vi "im_controller.vi"(6 "Reset":bool, 7 "Parameters":T1={"Stimulus"={"Type"=enum."Off", "Phase"=0.0, "Amplitude"=[0.0, 0.0, 0.0], "Injection point"=enum."Total pose", "Closed loop"=FALSE, "Offset"=[0.0, 0.0, 0.0], "Tip -> world"=TRUE, "Frequency"=0.0, "Length"=0.0}, "Goal Filter A"={"Speedup max"=0.0, "Speedup thresh"=0.15, "Speedup nonlin"=0.0, "Filters"=[]}, "Mode controls"={"Hold"=FALSE, "Cancellation"=FALSE, "Goal filter"=FALSE, "Trigger"=FALSE}, "Manipulator type"=enum."Current piezo", "Manipulator calibration"={"Tool offsets"=[[-0.47364116, -0.25724307, -1.1087934], [0.29673597, -0.25864395, -1.0971603], [-0.04366469, 0.4463568, -1.1035515]], "Tip light calibration"=[[3.2813332, 0.23462732, 0.17832138, -8265.082], [-0.20249099, 2.693321, -0.28150028, -33565.66], [-0.1458117, 0.68216485, 0.8833545, 26862.188], [-1.1202011e-18, 5.861468e-19, 1.7601345e-18, 1.0]], "Handle light calibration"=[[0.0, 0.0, 36200.0]], "Base pivots"=[], "Output pivots"=[[0.0, 0.0, -11360.0]], "Length center"=0.0, "Workspace height"=[], "Workspace diameter"=[0.0, 0.0, 36200.0], "Linearization"=[[0.0, 0.0, 36200.0]], "Stack travel"=400.0, "Saturation pos"=375.0, "Inverse filters"=[]}, "Network"={"Remote Host"="", "Send Status"=FALSE, "Send Port"=50, "Recv Commands"=FALSE, "Recv Port"=0}, "Goal Filter B"={"Speedup max"=0.0, "Speedup thresh"=0.0, "Speedup nonlin"=0.0, "Filters"=[]}, "Cancellation"={"KP"={"XY"=0.0, "Rxy"=0.0, "Z"=0.0, "Rz"=0.0}, "KI"=2.0, "KD"={"XY"=0.0, "Rxy"=0.0, "Z"=0.0, "Rz"=0.0}, "Max vel"=20.0, "Max acc"=61557.0, "Int error limit"=2.0, "RCM gain"=1.0, "Bypass"=FALSE, "Degraded gain"=3.0}, "Transition time"=0.0, "Estimation"={"Link"={"Measure noise"=[], "Process noise"=[], "Alt process noise"=[], "Alt turnoff cycles"=20, "Innovation limit"=[], "Residue threshold"=0.0, "Enable"=FALSE}, "Handle"={"Measure noise"=[], "Process noise"=[], "State limits"=[], "Innovation limit"=[], "Prediction Lookahead"=0.0, "Enable"=FALSE}}} {"Transition time" format="%_3f"; "Cancellation"."Degraded gain" min=0 max=1 step=0.1 format="%#_3p"; "Cancellation"."RCM gain" min=0 max=1 step=0.1 format="%#_3p"; "Cancellation"."KD"."Rz" min=0 max=1 step=0.1 format="%#_3p"; "Cancellation"."KD"."Rxy" min=0 max=1 step=0.1 format="%#_3p"; "Cancellation"."KD"."Z" min=0 max=1 step=0.1 format="%#_3p"; "Cancellation"."KD"."XY" min=0 max=1 step=0.1 format="%#_3p"; "Cancellation"."KI" min=0 max=1 step=0.01 format="%#_3p"; "Cancellation"."KP"."Rz" min=0 max=1 step=0.1 format="%#_3p"; "Cancellation"."KP"."Rxy" min=0 max=1 step=0.1 format="%#_3p"; "Cancellation"."KP"."Z" min=0 max=1 step=0.1 format="%#_3p"; "Cancellation"."KP"."XY" min=0 max=1 step=0.1 format="%#_3p"; "Cancellation"."Max acc" format="%#_3p"; "Goal Filter B"."Filters"."V limit range" format="%_3p"; "Goal Filter B"."Filters"."V limit" format="%_3p"; "Goal Filter B"."Filters"."Upper Q" format="%_3f"; "Goal Filter B"."Filters"."Upper Fc" format="%_3p"; "Goal Filter B"."Filters"."Lower Q" format="%_3f"; "Goal Filter B"."Filters"."Scale factor" format="%_3f"; "Goal Filter B"."Filters"."Lower Fc" format="%_3p"; "Goal Filter B"."Speedup nonlin" format="%_3p"; "Goal Filter B"."Speedup thresh" format="%_3p"; "Goal Filter B"."Speedup max" format="%_3p"; "Manipulator calibration"."Saturation pos" format="%#.1f"; "Manipulator calibration"."Stack travel" format="%#.1f"; "Manipulator calibration"."Output pivots" format="%#_6f"; "Manipulator calibration"."Base pivots" format="%#_6f"; "Manipulator calibration"."Handle light calibration" format="%#.1f"; "Manipulator calibration"."Tip light calibration" format="%#.1f"; "Goal Filter A"."Filters"."V limit range" format="%_3p"; "Goal Filter A"."Filters"."V limit" format="%_3p"; "Goal Filter A"."Filters"."Upper Q" format="%_3f"; "Goal Filter A"."Filters"."Upper Fc" format="%_3p"; "Goal Filter A"."Filters"."Lower Q" format="%_3f"; "Goal Filter A"."Filters"."Scale factor" format="%_3f"; "Goal Filter A"."Filters"."Lower Fc" format="%_3p"; "Goal Filter A"."Speedup nonlin" format="%_3p"; "Goal Filter A"."Speedup thresh" format="%_3p"; "Goal Filter A"."Speedup max" format="%_3p"; "Stimulus"."Length" min=0.0 max=100.0 step=100.0 format="%#_4p"; "Stimulus"."Frequency" min=0.0 step=100.0 format="%#_4g"; "Stimulus"."Offset" format="%#_3p"; "Stimulus"."Amplitude" format="%#_3p"; "Stimulus"."Phase" min=-180.0 max=360.0 step=100.0 format="%#.2f"}, 8 "Manipulator status":sgl[](array[numeric]), 10 "Stack error in":sgl[](array[numeric])) -> (4 "Saturation":bool, 5 "Output":sgl[](array[numeric]))   [LabVIEW 2013]
uses:
  testing/injection_point.ctl
  testing/stimulus.ctl
  testing/mode_conrols.ctl
  testing/Micron params.ctl
  asap/labview/testing/probe_calibration.ctl
  host/network_params.ctl
  testing/manipulator_cal.ctl
  filtering/goal_loop_parms.ctl
  decoupled_gain.ctl
  sq_control_params.ctl
  estimation_controls.ctl
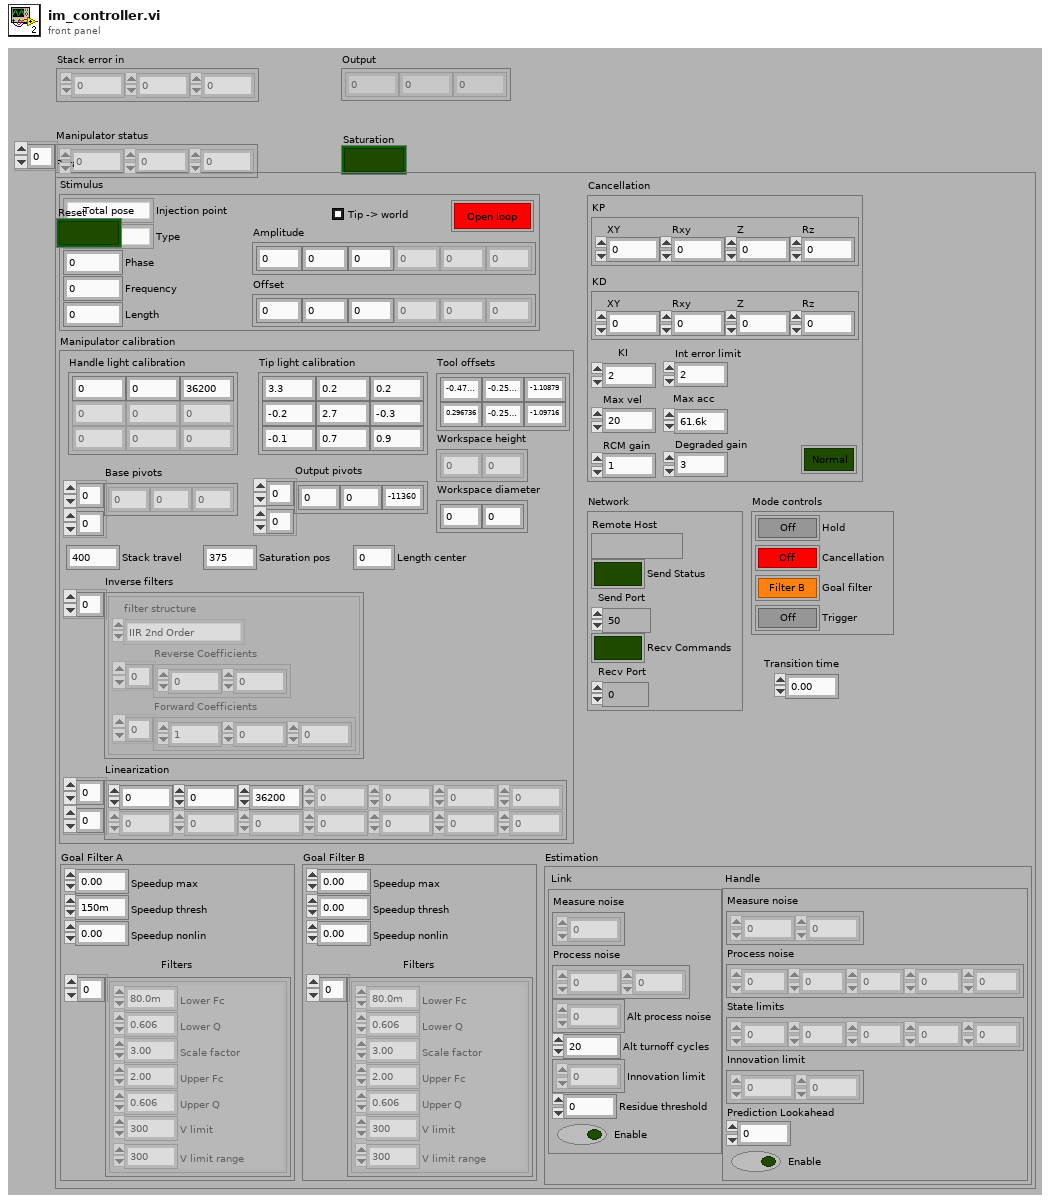
[diagram p1: front panel]
types:
  T1 = typedef "Micron params.ctl" = cluster{"Stimulus":T2, "Goal Filter A":T4, "Mode controls":T5, "Manipulator type":enum16{"Current piezo", "Voltage piezo"}, "Manipulator calibration":T6, "Network":T8, "Goal Filter B":T4, "Cancellation":T9, "Transition time":sgl, "Estimation":T11}
  T2 = typedef "stimulus.ctl" = cluster{"Type":enum16{"Off", "Step", "Sine", "Triangle", "Arbitrary"}, "Phase":dbl, "Amplitude":sgl[], "Injection point":T3, "Closed loop":bool, "Offset":sgl[], "Tip -> world":bool, "Frequency":dbl, "Length":dbl}
  T3 = typedef "injection_point.ctl" = enum16{"Total pose", "V limiter", "Goal ", "Link position", "KF link position", "Inverse kin", "Link goal", "Link error", "Controller", "Output", "Drive", "Light"}
  T4 = typedef "goal_loop_parms.ctl" = cluster{"Speedup max":sgl, "Speedup thresh":sgl, "Speedup nonlin":sgl, "Filters":cluster{"Lower Fc":sgl, "Lower Q":sgl, "Scale factor":sgl, "Upper Fc":sgl, "Upper Q":sgl, "V limit":sgl, "V limit range":sgl}[]}
  T5 = typedef "mode_conrols.ctl" = cluster{"Hold":bool, "Cancellation":bool, "Goal filter":bool, "Trigger":bool}
  T6 = typedef "manipulator_cal.ctl" = cluster{"Tool offsets":sgl[][], "Tip light calibration":T7, "Handle light calibration":T7, "Base pivots":sgl[][], "Output pivots":sgl[][], "Length center":sgl, "Workspace height":sgl[], "Workspace diameter":sgl[], "Linearization":sgl[][], "Stack travel":sgl, "Saturation pos":sgl, "Inverse filters":cluster{"filter structure":enum32{"IIR 2nd Order", "IIR 4th Order"}, "Reverse Coefficients":dbl[], "Forward Coefficients":dbl[]}[]}
  T7 = typedef "probe_calibration.ctl" = sgl[][]
  T8 = typedef "network_params.ctl" = cluster{"Remote Host":string, "Send Status":bool, "Send Port":u16, "Recv Commands":bool, "Recv Port":u16}
  T9 = typedef "sq_control_params.ctl" = cluster{"KP":T10, "KI":sgl, "KD":T10, "Max vel":sgl, "Max acc":sgl, "Int error limit":sgl, "RCM gain":sgl, "Bypass":bool, "Degraded gain":sgl}
  T10 = typedef "decoupled_gain.ctl" = cluster{"XY":sgl, "Rxy":sgl, "Z":sgl, "Rz":sgl}
  T11 = typedef "estimation_controls.ctl" = cluster{"Link":cluster{"Measure noise":dbl[], "Process noise":dbl[], "Alt process noise":dbl[], "Alt turnoff cycles":i32, "Innovation limit":dbl[], "Residue threshold":dbl, "Enable":bool}, "Handle":cluster{"Measure noise":dbl[], "Process noise":dbl[], "State limits":dbl[], "Innovation limit":dbl[], "Prediction Lookahead":sgl, "Enable":bool}}
  T12 = cluster{"XY":dbl, "Rxy":dbl, "Z":dbl, "Rz":dbl}[]
  T13 = cluster{"XY":bool, "Rxy":bool, "Z":bool, "Rz":bool}[]
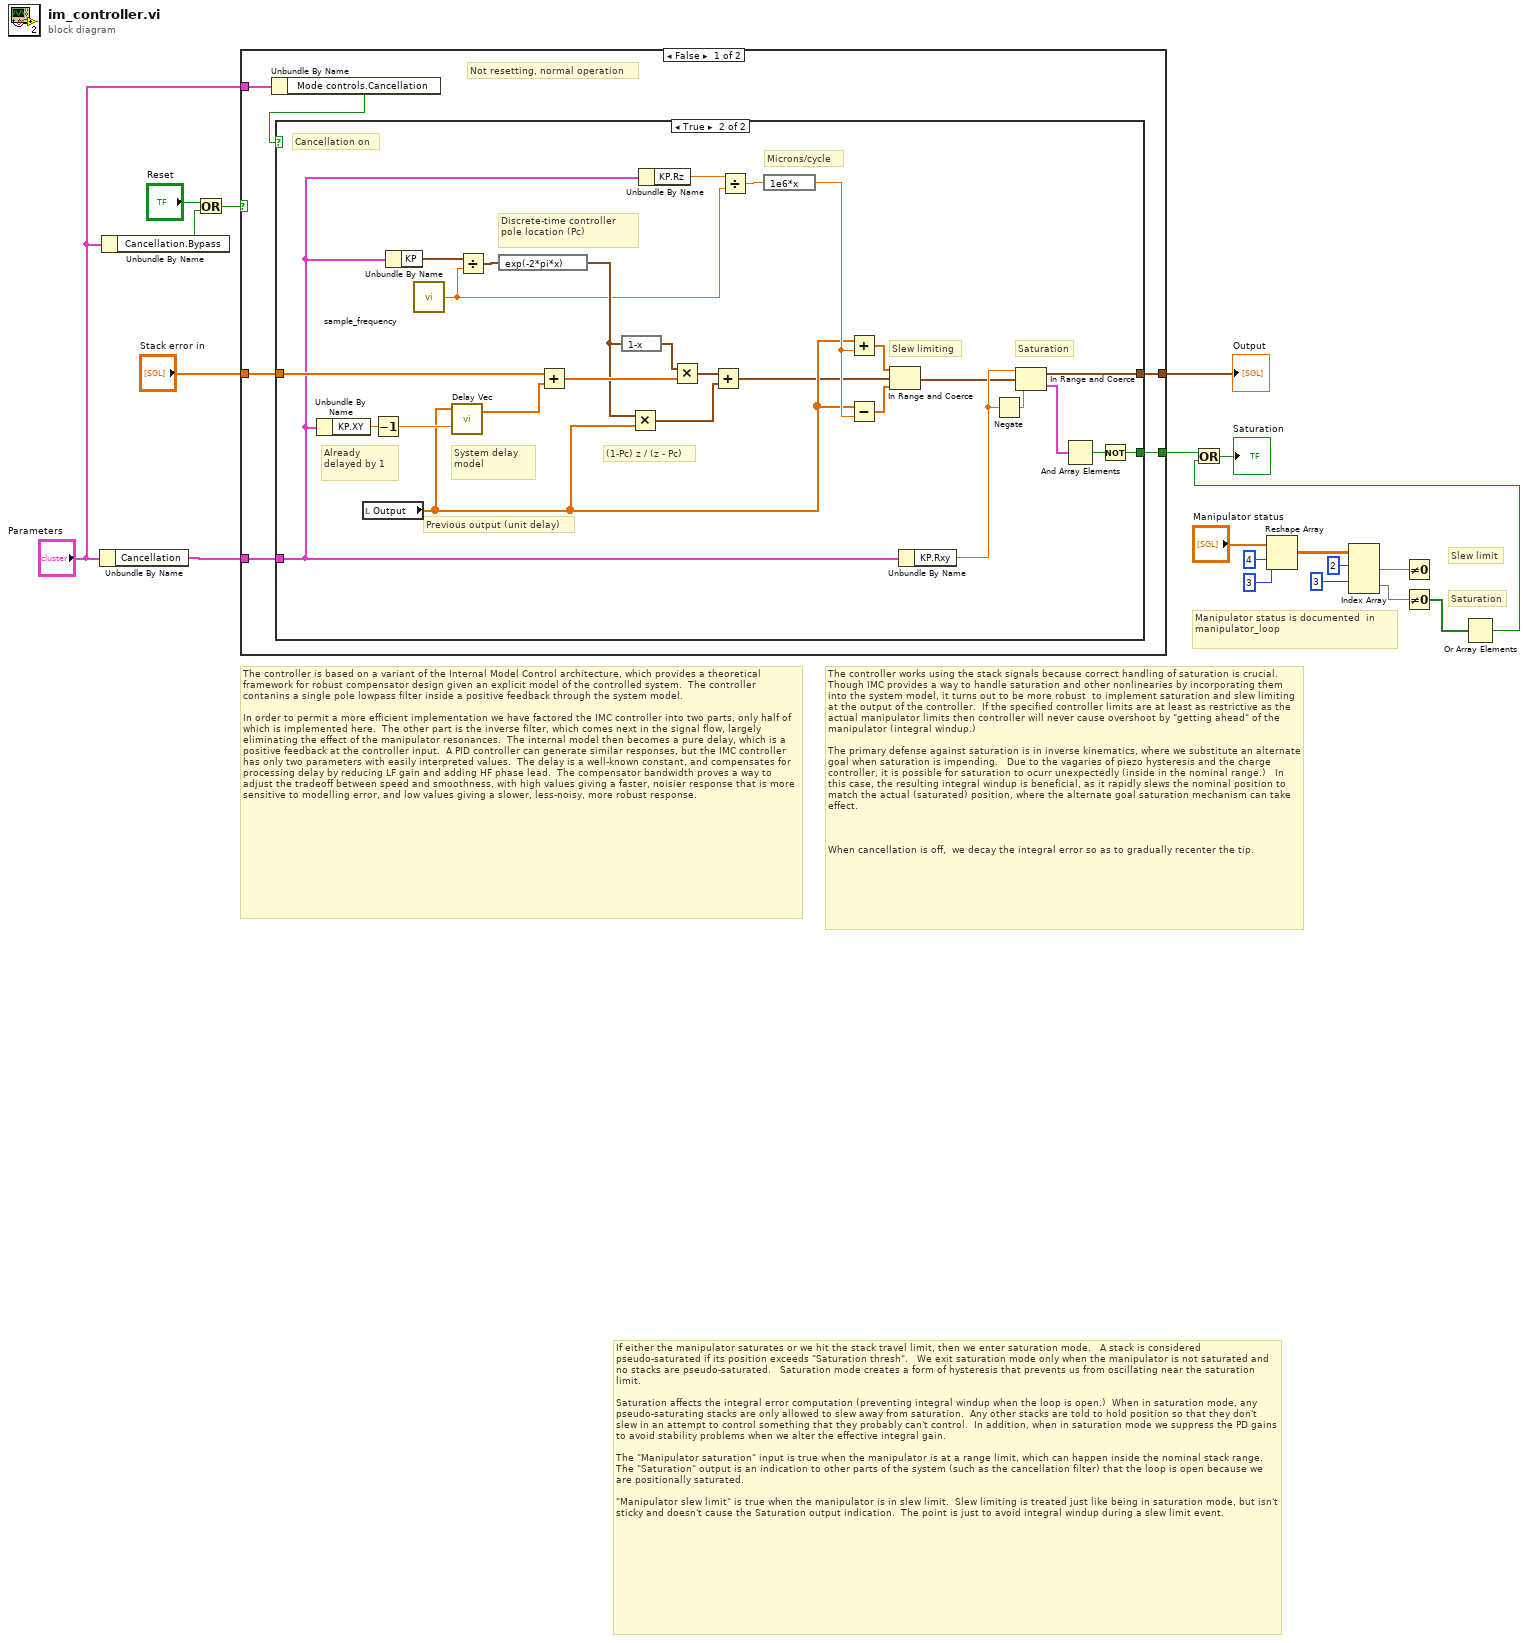
[diagram p0: block diagram]
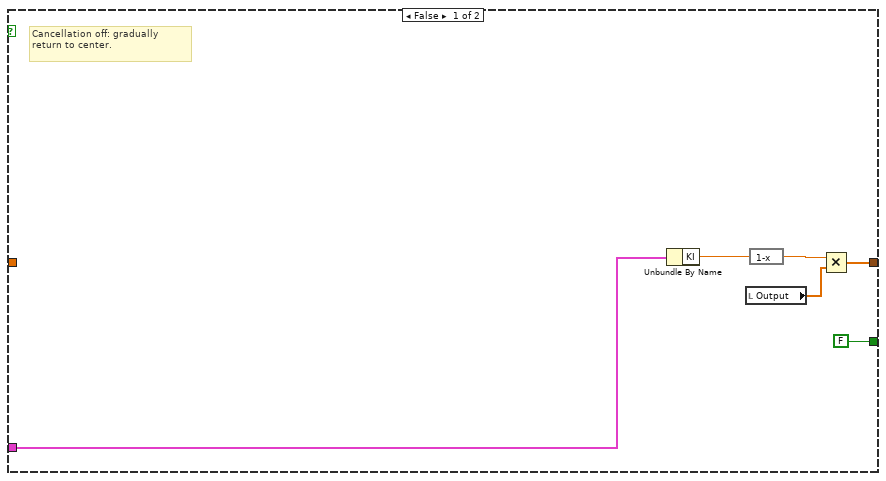
[diagram p2: hidden frame]
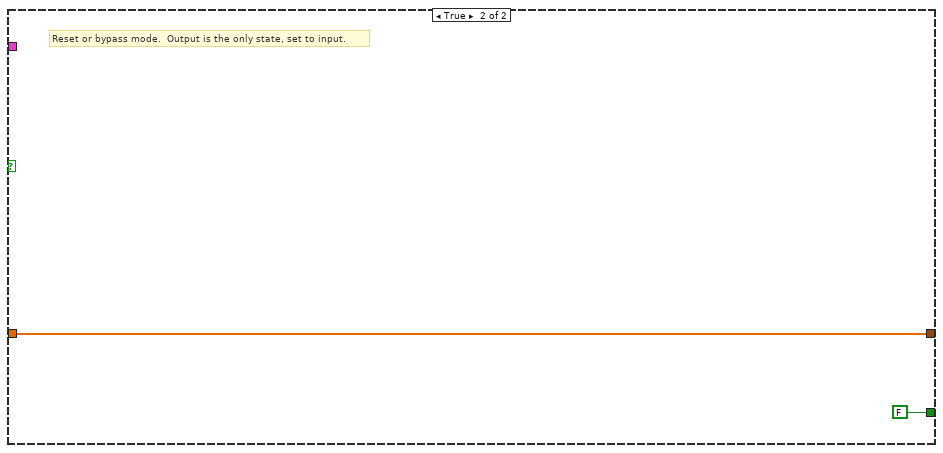
[diagram p3: hidden frame]
diagram:
  # "The controller works using the stack signals because correct handling of saturation is crucial.  Though IMC provides a way to handle saturation and other nonlinearies by incorporating them into the system model, it turns out to be more robust  to implement saturation and slew limiting at the output of the controller.  If the specified controller limits are at least as restrictive as the actual manipulator limits then controller will never cause overshoot by \"getting ahead\" of the manipulator (integral windup.)\n\nThe primary defense against saturation is in inverse kinematics, where we substitute an alternate goal when saturation is impending.   Due to the vagaries of piezo hysteresis and the charge controller, it is possible for saturation to ocurr unexpectedly (inside in the nominal range.)   In this case, the resulting integral windup is beneficial, as it rapidly slews the nominal position to match the actual (saturated) position, where the alternate goal saturation mechanism can take effect.\n\n\n\nWhen cancellation is off,  we decay the integral error so as to gradually recenter the tip."
  # "Saturation"
  # "Slew limit"
  # "Manipulator status is documented  in manipulator_loop"
  # "If either the manipulator saturates or we hit the stack travel limit, then we enter saturation mode.   A stack is considered pseudo-saturated if its position exceeds \"Saturation thresh\".   We exit saturation mode only when the manipulator is not saturated and no stacks are pseudo-saturated.   Saturation mode creates a form of hysteresis that prevents us from oscillating near the saturation limit.  \n\nSaturation affects the integral error computation (preventing integral windup when the loop is open.)  When in saturation mode, any  pseudo-saturating stacks are only allowed to slew away from saturation.  Any other stacks are told to hold position so that they don't slew in an attempt to control something that they probably can't control.  In addition, when in saturation mode we suppress the PD gains to avoid stability problems when we alter the effective integral gain.\n\nThe \"Manipulator saturation\" input is true when the manipulator is at a range limit, which can happen inside the nominal stack range. The \"Saturation\" output is an indication to other parts of the system (such as the cancellation filter) that the loop is open because we are positionally saturated.  \n\n\"Manipulator slew limit\" is true when the manipulator is in slew limit.  Slew limiting is treated just like being in saturation mode, but isn't sticky and doesn't cause the Saturation output indication.  The point is just to avoid integral windup during a slew limit event."
  # "The controller is based on a variant of the Internal Model Control architecture, which provides a theoretical framework for robust compensator design given an explicit model of the controlled system.  The controller contanins a single pole lowpass filter inside a positive feedback through the system model.\n\nIn order to permit a more efficient implementation we have factored the IMC controller into two parts, only half of which is implemented here.  The other part is the inverse filter, which comes next in the signal flow, largely eliminating the effect of the manipulator resonances.  The internal model then becomes a pure delay, which is a positive feedback at the controller input.  A PID controller can generate similar responses, but the IMC controller has only two parameters with easily interpreted values.  The delay is a well-known constant, and compensates for processing delay by reducing LF gain and adding HF phase lead.  The compensator bandwidth proves a way to adjust the tradeoff between speed and smoothness, with high values giving a faster, noisier response that is more sensitive to modelling error, and low values giving a slower, less-noisy, more robust response."
  n1 = Unbundle By Name("Parameters") -> ("Cancellation"=w2:T9)
  n2 = Unbundle By Name("Parameters") -> ("Cancellation.Bypass"=w4:bool)
  n3 = Or(x="Reset", y=w4) -> (x .or. y?=w6:bool)
  n4 = case shown="False" w6 {
    tunnel: "Parameters" -> [w25 _]
    tunnel: "Stack error in" -> [w24 w60]
    tunnel: w2 -> [w23 _]
    tunnel: [w22 w60] -> w18
    tunnel: [w20 FALSE] -> w11
    frame False {
      # "Not resetting, normal operation"
      n5 = Unbundle By Name(w25) -> ("Mode controls.Cancellation"=w21:bool)
      n6 = case shown="True" w21 {
        tunnel: [w26 w42] -> w22
        tunnel: [FALSE w56] -> w20
        tunnel: w24 -> [_ w53]
        tunnel: w23 -> [w27 w41]
        frame False {
          # "Cancellation off: gradually return to center."
          n7 = Unbundle By Name(w27) -> ("KI"=w31:sgl)
          n8 = local read "Output"() -> (w28:sgl[])
          n9 = expression code="1-x"(w31) -> (w30:sgl)
          n10 = Multiply(x=w30, y=w28) -> (x*y=w26:sgl[])
        }
        frame True {
          # "System delay model"
          # "Saturation"
          # "Slew limiting"
          # "Microns/cycle"
          # "(1-Pc) z / (z - Pc)"
          # "Already delayed by 1"
          # "Previous output (unit delay)"
          # "Discrete-time controller pole location (Pc)"
          # "Cancellation on"
          n11 = Unbundle By Name(w41) -> ("KP.XY"=w45:sgl)
          n12 = local read "Output"() -> (w33:sgl[])
          n13 = Decrement(x=w45) -> (x-1=w54:sgl)
          n14 = Unbundle By Name(w41) -> ("KP"=w44:T10)
          n15 = call "sample_frequency.vi"() -> ("Sample frequency"=w39:dbl)
          n16 = call "Delay Vec.vi"("Delay length"=w54, "X"=w33) -> ("Delayed X"=w52:sgl[])  [unwired: 1 in, 2 out]
          n17 = Divide(x=w44, y=w39) -> (x/y=w55:cluster{"XY":dbl, "Rxy":dbl, "Z":dbl, "Rz":dbl})
          n18 = expression code="exp(-2*pi*x)"(w55) -> (w49:cluster{"XY":dbl, "Rxy":dbl, "Z":dbl, "Rz":dbl})
          n19 = Add(x=w53, y=w52) -> (x+y=w51:sgl[])
          n20 = expression code="1-x"(w49) -> (w50:cluster{"XY":dbl, "Rxy":dbl, "Z":dbl, "Rz":dbl})
          n21 = Multiply(x=w49, y=w33) -> (x*y=w47:cluster{"XY":dbl, "Rxy":dbl, "Z":dbl, "Rz":dbl})
          n22 = Unbundle By Name(w41) -> ("KP.Rz"=w40:sgl)
          n23 = Multiply(x=w50, y=w51) -> (x*y=w48:cluster{"XY":dbl, "Rxy":dbl, "Z":dbl, "Rz":dbl})
          n24 = Add(x=w48, y=w47) -> (x+y=w32:cluster{"XY":dbl, "Rxy":dbl, "Z":dbl, "Rz":dbl})
          n25 = Divide(x=w40, y=w39) -> (x/y=w38:dbl)
          n26 = expression code="1e6*x"(w38) -> (w36:dbl)
          n27 = Add(x=w33, y=w36) -> (x+y=w34:dbl[])
          n28 = Subtract(x=w33, y=w36) -> (x-y=w37:dbl[])
          n29 = In Range and Coerce(upper limit=w34, x=w32, lower limit=w37) -> (coerced(x)=w35:T12)  [unwired: 1 out]
          n30 = Unbundle By Name(w41) -> ("KP.Rxy"=w43:sgl)
          n31 = Negate(x=w43) -> (-x=w58:sgl)
          n32 = In Range and Coerce(upper limit=w43, x=w35, lower limit=w58) -> (coerced(x)=w42:T12, In Range?=w46:T13)
          n33 = And Array Elements(Boolean array=w46) -> (logical AND=w57:bool)
          n34 = Not(x=w57) -> (.not. x?=w56:bool)
        }
      }
    }
    frame True {
      # "Reset or bypass mode.  Output is the only state, set to input."
    }
  }
  "Output" <- w18
  n35 = Reshape Array("Manipulator status", 4 ("dimension size"), 3 ("dimension size")) -> (w15:sgl[][])
  n36 = Index Array(array=w15, index (row) #1=2 ("index (row)"), index (row) #2=3 ("index (row)")) -> (element #1=w16:sgl[], element #2=w17:sgl[])  [unwired: 2 in]
  n37 = Not Equal To 0?(x=w16) -> ()  [unwired: 1 out]
  n38 = Not Equal To 0?(x=w17) -> (x != 0?=w7:bool[])
  n39 = Or Array Elements(Boolean array=w7) -> (logical OR=w10:bool)
  n40 = Or(x=w11, y=w10) -> (x .or. y?=→"Saturation":bool)
